vi "Read Shutter Mode.vi"(8 "error in (no error)":errorcluster, 11 "CCDCamera in":refnum<class "Simulated_CCD_Camera.lvclass">) -> (0 "error out":errorcluster, 2 "Shutter Mode":u8(ring)=2 items=["Fully Auto", "OPEN", "CLOSED"], 3 "CCDCamera out":refnum<class "Simulated_CCD_Camera.lvclass">)   [LabVIEW 2018, in "Simulated_CCD_Camera.lvclass"]
uses:
  Simulated_CCD_Camera.lvclass
  Simulated_CCD_Camera.lvclass/Simulated_CCD_Camera.ctl
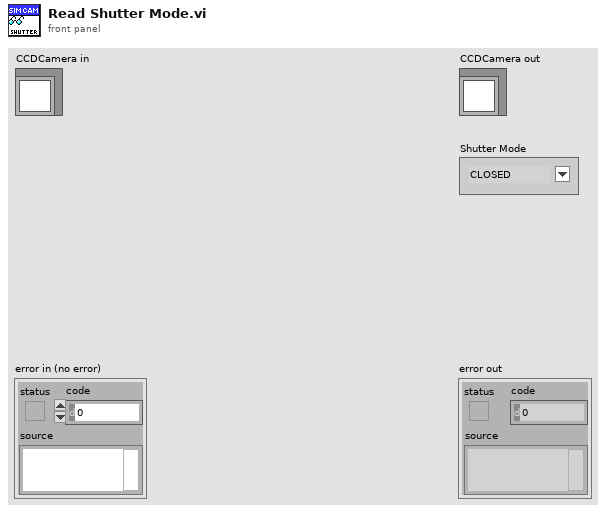
[diagram p1: front panel]
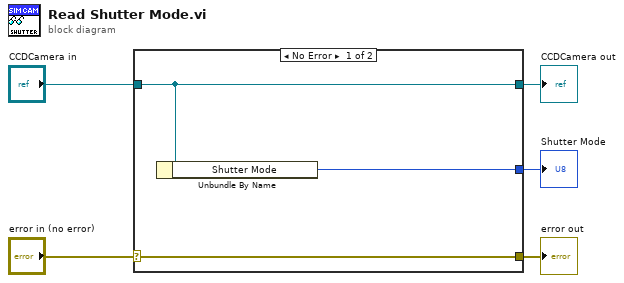
[diagram p0: block diagram]
diagram:
  n1 = case shown="No Error" "error in (no error)" {
    selector: "error in (no error)" -> [w8 w9]
    tunnel: [w8 w9] -> w4
    tunnel: [w7 w10] -> w2
    tunnel: "CCDCamera in" -> [w7 w10]
    tunnel: [w6 _] -> w1
    frame No Error {
      n2 = Unbundle By Name(w7) -> ("Shutter Mode"=w6:u8)
    }
    frame Error {
    }
  }
  "error out" <- w4
  "CCDCamera out" <- w2
  "Shutter Mode" <- w1
